vi "test Get Port Number.vi"(8 "error in":errorcluster, 11 "TestCase in":refnum<class "Scripting.lvclass">) -> (0 "error out":errorcluster, 3 "TestCase out":refnum<class "Scripting.lvclass">)   [LabVIEW 2024, in "Scripting.lvclass"]
uses:
  Scripting.lvclass
  Shared/Direction.ctl
  Shared/Transfer Speed.ctl
  Scripting.lvclass/Scripting.ctl
  <vilib>/addons/_JKI Toolkits/VI Tester/TestCase.llb/TestCase.lvclass
  Scripting/AIM/AIM ARINC 429 Scripting.lvlib
  C:/Program Files/National Instruments/LabVIEW 2024/vi.lib/addons/_JKI Toolkits/VI Tester/TestCase.llb/TestCase.lvclass
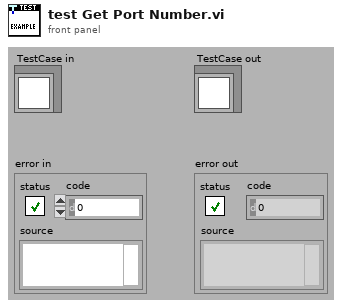
[diagram p1: front panel]
types:
  T1 = typedef "Transfer Speed.ctl" = enum16{"LO (12.5 kb/s)", "HI (100 kb/s)"}
  T2 = typedef "Direction.ctl" = enum16{"Rx", "Tx"}
  T3 = typedef "Custom Device API.lvlib/Custom Device Item Ref.ctl" = u64
  T4 = cluster{"channel":u8, "direction":T2, "speed":T1}
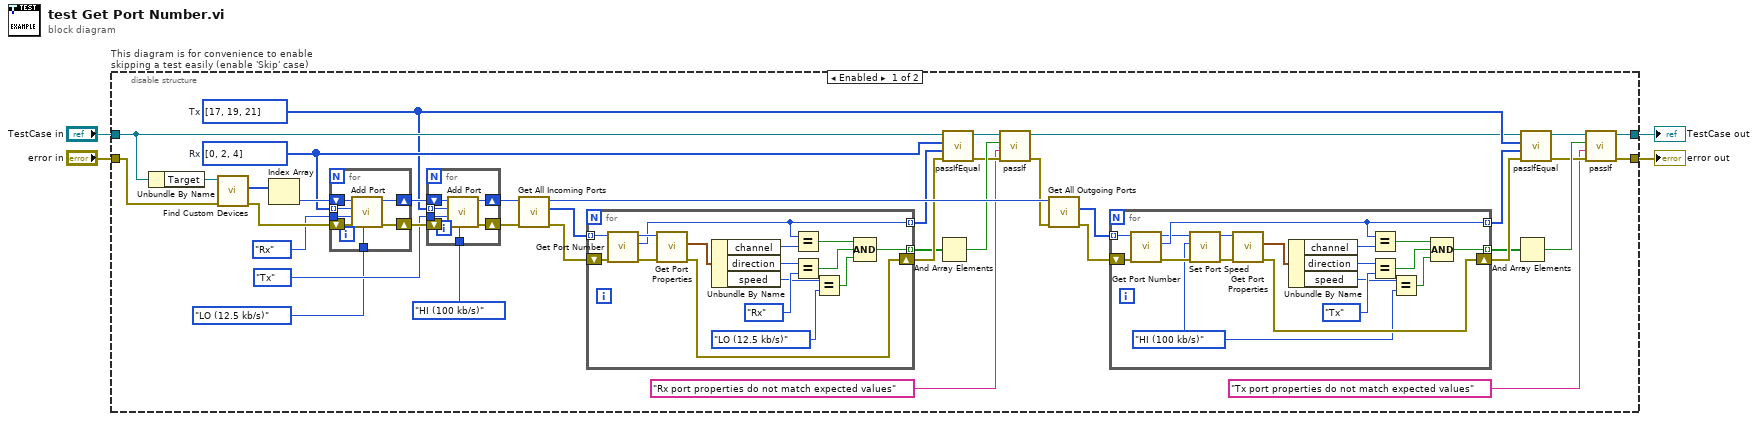
[diagram p0: block diagram]
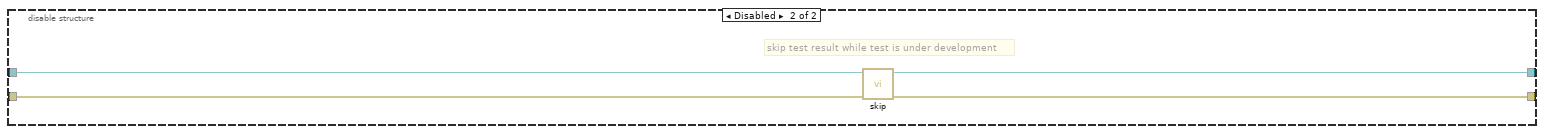
[diagram p2: hidden frame]
diagram:
  n1 = disable-structure "This diagram is for convenience to enable skipping a test easily (enable 'Skip' case)" shown="Enabled" {
    disable-tunnel: "TestCase in" -> [w42 w95]
    disable-tunnel: [w9 w93] -> w1
    disable-tunnel: [w10 w94] -> w3
    disable-tunnel: "error in" -> [w36 w92]
    frame Enabled {
      w27 = u16[] [17, 19, 21]  # Tx
      w28 = u16[] [0, 2, 4]  # Rx
      n2 = Unbundle By Name(w42) -> ("Target"=w43:refnum<k24>)
      n3 = call "Find Custom Devices.vi"("error in"=w36, "target"=w43) -> ("error out"=w33:errorcluster, "AIM ARINC 429 custom devices"=w35:T3[])  [unwired: 7 in, 1 out]
      n4 = Index Array(array=w35) -> (element=w34:T3)  [unwired: 1 in]
      n5 = for {
        shift-right: [w73] -> w32
        shift-left: w34 -> [w75]
        shift-right: [w72] -> w31
        shift-left: w33 -> [w74]
        tunnel: Direction."Rx" ("direction") -> [w71]
        tunnel: w28 -> [w70] mode=indexing
        tunnel: Transfer_Speed."LO (12.5 kb/s)" ("speed") -> [w69]
        n6 = call "Add Port.vi"("speed"=w69, "error in"=w74, "direction"=w71, "port number"=w70, "custom device ref"=w75) -> ("error out"=w72:errorcluster, "custom device ref out"=w73:T3)  [unwired: 4 in, 1 out]
      }
      n7 = for {
        shift-right: [w66] -> w26
        shift-left: w31 -> [w67]
        shift-right: [w65] -> w25
        shift-left: w32 -> [w68]
        tunnel: Direction."Tx" ("direction") -> [w64]
        tunnel: w27 -> [w63] mode=indexing
        tunnel: Transfer_Speed."HI (100 kb/s)" ("speed") -> [w62]
        n8 = call "Add Port.vi"("speed"=w62, "error in"=w67, "direction"=w64, "port number"=w63, "custom device ref"=w68) -> ("error out"=w66:errorcluster, "custom device ref out"=w65:T3)  [unwired: 4 in, 1 out]
      }
      n9 = call "Get All Incoming Ports.vi"("error in"=w26, "custom device ref"=w25) -> ("error out"=w40:errorcluster, "incoming ports"=w39:T3[], "custom device ref out"=w41:T3)  [unwired: 7 in]
      n10 = for {
        tunnel: w39 -> [w90] mode=indexing
        shift-right: [w86] -> w37
        shift-left: w40 -> [w91]
        tunnel: [w84] -> w38 mode=indexing
        tunnel: [w76] -> w24 mode=indexing
        n11 = call "Get Port Number.vi"("error in"=w91, "port ref"=w90) -> ("error out"=w89:errorcluster, "port number"=w84:u16, "port ref out"=w88:T3)  [unwired: 6 in, 1 out]
        n12 = call "Get Port Properties.vi"("error in"=w89, "port ref"=w88) -> ("error out"=w86:errorcluster, "channel configuration"=w87:T4)  [unwired: 6 in, 2 out]
        n13 = Unbundle By Name(w87) -> ("channel"=w85:u8, "direction"=w83:T2, "speed"=w81:T1)
        n14 = Equal?(x=w84, y=w85) -> (x = y?=w79:bool)
        n15 = Equal?(x=w83, y=Direction."Rx") -> (x = y?=w78:bool)
        n16 = Equal?(x=w81, y=Transfer_Speed."LO (12.5 kb/s)") -> (x = y?=w77:bool)
        n17 = Compound Arithmetic op=AND(w79, w78, w77) -> (w76:bool)
      }
      n18 = And Array Elements(Boolean array=w24) -> (logical AND=w23:bool)
      n19 = call-dynamic "passIfEqual.vi"("error in (no error)"=w37, "y"=w38, "x"=w28, "TestCase in"=w42) -> ("error out"=w22:errorcluster, "TestCase out"=w20:refnum<class "Scripting.lvclass">)  [unwired: 6 in]
      n20 = call-dynamic "passIf.vi"("error in (no error)"=w22, "message (\"\")"="Rx port properties do not match expected values" ("message (\"\")"), "pass"=w23, "TestCase in"=w20) -> ("error out"=w21:errorcluster, "TestCase out"=w19:refnum<class "Scripting.lvclass">)  [unwired: 6 in]
      n21 = call "Get All Outgoing Ports.vi"("error in"=w21, "custom device ref"=w41) -> ("error out"=w18:errorcluster, "outgoing ports"=w17:T3[])  [unwired: 7 in, 1 out]
      n22 = for {
        tunnel: w17 -> [w60] mode=indexing
        shift-right: [w58] -> w15
        shift-left: w18 -> [w61]
        tunnel: [w56] -> w16 mode=indexing
        tunnel: [w49] -> w13 mode=indexing
        w44 = Transfer_Speed."HI (100 kb/s)" ("y")
        n23 = call "Get Port Number.vi"("error in"=w61, "port ref"=w60) -> ("error out"=w46:errorcluster, "port number"=w56:u16, "port ref out"=w48:T3)  [unwired: 6 in, 1 out]
        n24 = call "Set Port Speed.vi"("error in"=w46, "speed"=w44, "port ref"=w48) -> ("error out"=w45:errorcluster, "port ref out"=w47:T3)  [unwired: 7 in]
        n25 = call "Get Port Properties.vi"("error in"=w45, "port ref"=w47) -> ("error out"=w58:errorcluster, "channel configuration"=w59:T4)  [unwired: 6 in, 2 out]
        n26 = Unbundle By Name(w59) -> ("channel"=w57:u8, "direction"=w55:T2, "speed"=w53:T1)
        n27 = Equal?(x=w56, y=w57) -> (x = y?=w52:bool)
        n28 = Equal?(x=w55, y=Direction."Tx") -> (x = y?=w51:bool)
        n29 = Equal?(x=w53, y=w44) -> (x = y?=w50:bool)
        n30 = Compound Arithmetic op=AND(w52, w51, w50) -> (w49:bool)
      }
      n31 = And Array Elements(Boolean array=w13) -> (logical AND=w14:bool)
      n32 = call-dynamic "passIfEqual.vi"("error in (no error)"=w15, "y"=w16, "x"=w27, "TestCase in"=w19) -> ("error out"=w11:errorcluster, "TestCase out"=w12:refnum<class "Scripting.lvclass">)  [unwired: 6 in]
      n33 = call-dynamic "passIf.vi"("error in (no error)"=w11, "message (\"\")"="Tx port properties do not match expected values" ("message (\"\")"), "pass"=w14, "TestCase in"=w12) -> ("error out"=w10:errorcluster, "TestCase out"=w9:refnum<class "Scripting.lvclass">)  [unwired: 6 in]
    }
    frame Disabled {
      # "skip test result while test is under development"
      n34 = call <vilib>:"skip.vi"("error in (no error)"=w92, "TestCase in"=w95) -> ("error out"=w94:errorcluster, "TestCase out"=w93:refnum<class "Scripting.lvclass">)  [unwired: 8 in]
    }
  }
  "error out" <- w3
  "TestCase out" <- w1
